vi "导出数据.vi"(8 "error in (no error)":errorcluster caption="错误输入（无错误）", 9 "text data":string[][](array[string]) caption="数据", 10 "column headers":string[](array[string]) caption="列名", 11 "path":path caption="路径") -> (0 "error out":errorcluster caption="错误输出")   [LabVIEW 2020]
uses:
  <vilib>/Utility/NIReport.llb/Report Type.ctl
  <vilib>/Utility/NIReport.llb/Append Text Table to Report (wrap).vi
  <vilib>/Utility/NIReport.llb/NI_report.lvclass
  <vilib>/Utility/NIReport.llb/NI_ReportGenerationCore.lvlib
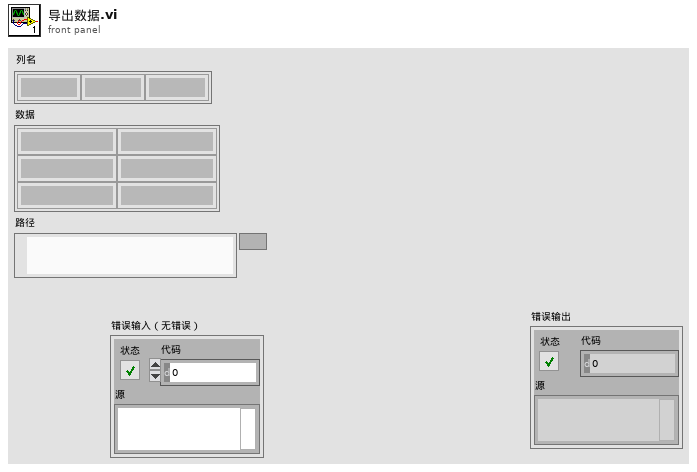
[diagram p1: front panel]
types:
  T1 = cluster{"position (excel)":cluster{"row":i32, "column":i32}, "name (excel)":string, "bookmark (word)":string}
  T2 = enum16{"maximized", "minimized", "normal", "no change"}
  T3 = typedef "NI_ReportGenerationCore.lvlib/Report Type.ctl" = enum16{"HTML", "Word", "Excel"}
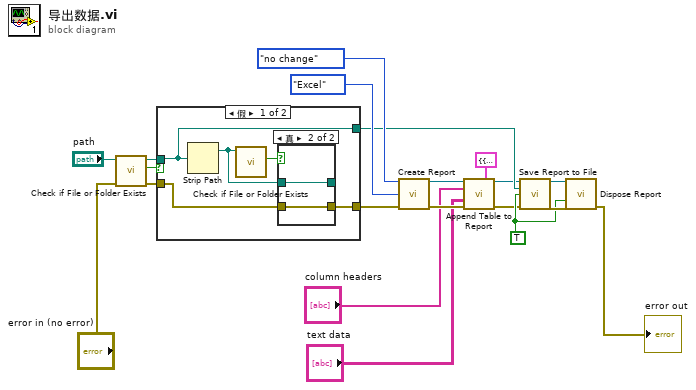
[diagram p0: block diagram]
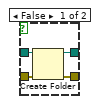
[diagram p2: hidden frame]
diagram:
  w11 = TRUE ("prompt to replace? (F)")
  n1 = call <vilib>:"Check if File or Folder Exists.vi"("error in (no error)"="error in (no error)", "path"="path") -> ("error out"=w19:errorcluster, "file or folder exists?"=w20:bool, "dup path"=w18:path)  [unwired: 7 in]
  n2 = case shown="假" w20 {
    tunnel: w19 -> [w25 w33]
    tunnel: w18 -> [w21 w32]
    tunnel: [w22 w33] -> w15
    tunnel: [w21 w32] -> w12
    frame False {
      n3 = Strip Path(path=w21) -> (stripped path=w24:path)  [unwired: 1 out]
      n4 = call <vilib>:"Check if File or Folder Exists.vi"("path"=w24) -> ("file or folder exists?"=w23:bool)  [unwired: 8 in, 2 out]
      n5 = case shown="真" w23 {
        tunnel: w25 -> [w29 w31]
        tunnel: [w28 w31] -> w22
        tunnel: w24 -> [w27 w30]
        tunnel: [w26 w30] -> _
        frame False {
          n6 = Create Folder(path (use dialog)=w27, error in=w29) -> (created path=w26:path, error out=w28:errorcluster)  [unwired: 1 in, 1 out]
        }
        frame True {
        }
      }
    }
    frame True {
    }
  }
  n7 = call <vilib>:"Create Report.vi"("window state (normal)"=T2."no change", "report type"=Report_Type."Excel", "error in (no error)"=w15) -> ("report out"=w9:refnum<class "NI_report.lvclass">, "error out"=w7:errorcluster)  [unwired: 11 in]
  n8 = call-poly <vilib>:"Append Table to Report.vi"("report in"=w9, "MS Office parameters"=T1 {"position (excel)"={"row"=0, "column"=0}, "name (excel)"="", "bookmark (word)"=""}, "column headers"="column headers", "text data"="text data", "error in (no error)"=w7) -> ("report out"=w8:refnum<class "NI_report.lvclass">, "error out"=w6:errorcluster)  [unwired: 7 in, 2 out]
  n9 = call-dynamic "Save Report to File.vi"("report in"=w8, "report file path"=w12, "prompt to replace? (F)"=w11, "error in (no error)"=w6) -> ("report out"=w14:refnum<class "NI_report.lvclass">, "error out"=w13:errorcluster)  [unwired: 10 in]
  n10 = call-dynamic "Dispose Report.vi"("report in"=w14, "save changes? (F)"=w11, "error in (no error)"=w13) -> ("error out"=→"error out":errorcluster)  [unwired: 12 in]
